vi "odd bit extractor(SubVI).vi"(10 "Loop Index":i8, 11 "input PN Sequence":i8[](array[numeric])) -> (3 "Odd bits":i8)   [LabVIEW 2026]
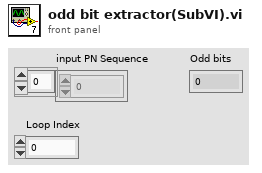
[diagram p1: front panel]
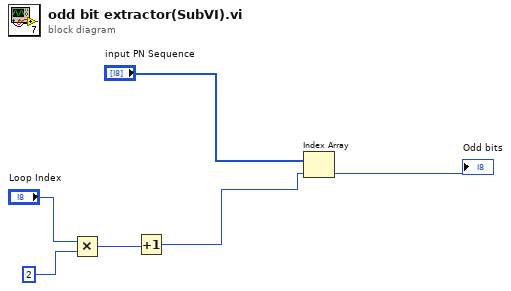
[diagram p0: block diagram]
diagram:
  n1 = Multiply(x="Loop Index", y=i8 2) -> (x*y=w4:i8)
  n2 = Increment(x=w4) -> (x+1=w5:i8)
  n3 = Index Array(array="input PN Sequence", index=w5) -> (element=→"Odd bits":i8)
